vi "UndeploySharedVariables.vi"(1 "Target IPAddress":string) -> (0 "error out":errorcluster)   [LabVIEW 2013]
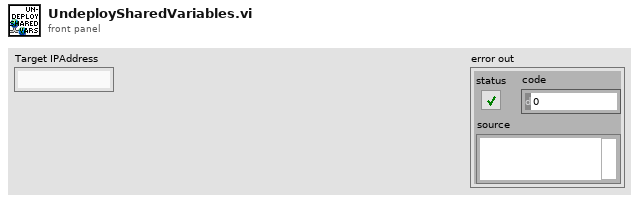
[diagram p1: front panel]
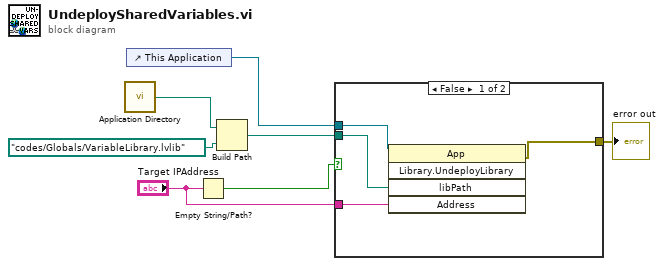
[diagram p0: block diagram]
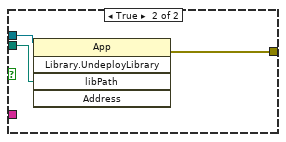
[diagram p2: hidden frame]
diagram:
  n1 = call <vilib>:"Application Directory.vi"() -> ("Application Directory"=w3:path)
  n2 = control-ref of="This Application"() -> (w5:refnum<vi>)
  n3 = Empty String/Path?(string/path="Target IPAddress") -> (empty?=w6:bool)
  n4 = Build Path(base path=w3, name or relative path=path "codes/Globals/VariableLibrary.lvlib" ("Path")) -> (appended path=w2:path)
  n5 = case shown="False" w6 {
    tunnel: "Target IPAddress" -> [w11 _]
    tunnel: w5 -> [w10 w14]
    tunnel: [w9 w13] -> w1
    tunnel: w2 -> [w8 w12]
    frame False {
      n6 = invoke class="App" method="Library.UndeployLibrary"(reference=w10, "libPath"=w8, "Address"=w11) -> (error out=w9:errorcluster)  [unwired: 2 in, 4 out]
    }
    frame True {
      n7 = invoke class="App" method="Library.UndeployLibrary"(reference=w14, "libPath"=w12) -> (error out=w13:errorcluster)  [unwired: 3 in, 4 out]
    }
  }
  "error out" <- w1
